vi "GEA2 Read and Update ERD.vi"(2 "Read Timeout (ms)":u32=500, 3 "Retry Count":i32=5, 5 "GEA Inputs":T2 {"Destination" format="%.0x"; "Source" format="%.0x"}, 7 "ERD Number":u16 format="%.0x", 9 "Update Information":string, 11 "Error In":errorcluster, 13 "Verify ERD Response?":bool=TRUE) -> (6 "Updated Raw Data Out":string, 8 "Updated ERD Data Out":T1 {"ERD Number" format="%.0x"}, 15 "Error Out":errorcluster)   [LabVIEW 2016, in "GEA2_Toolkit.lvlib"]
doc: "This VI reads and updates a single ERD based on the information provided in the Update information input. This VI only supports ERDs that support read and write capability. The update information should contain all of the bits that you wish to be updated in the ERD. Just specify the bits you want to update (ex. 0=1) and put whether or not you want them to be True (1) or False (0). You can specify a range of bits by using the - command in between two numbers (ex. 0-7=1 would change bits 0, 1, 2, 3, 4, 5, 6, 7 to true). The update information is converted to an array of strings by a comma delimiter. So, seperate your update information pieces by commas (Ex. if you wanted to make bits 0 and 10 false you could use the message: 0=0,10=0). Make sure you don't set the same bit twice or only the 2nd setting will ocurr (ex. 0=1,0=0 will only set bit 0 to false). If you were to write the following ERD data (00 01 02), byte 00 would be the byte 0 and contain bits 0-7, byte 01 would be byte 1 and contain bits 8-15, and byte 02 would be byte 2 and contain bits 16-23. For all bytes, the right-most bit is the first bit and the left-most bit is the last (Ex. For byte 00 being the hex value 0x01, bit 0 would be equal to 1 and would be the right-most bit (00000001)."
uses:
  library/GEA2_Toolkit.lvlib
  type defs/Source_Destination.ctl
  type defs/ERD Read Data Out.ctl
  C:/Technology Lab/NI-2010/Trunk/Utility/LabVIEW GEA2 Toolkit v1.0.0.0/Appliance.NET/GeaCommunication.dll
  Appliance.NET/GeaCommunication.dll
  type defs/ERD Read Data In.ctl
  type defs/Data Type.ctl
  type defs/ERD Write Data In.ctl
panel:
  out "GEA2 Reference Out":refnum<k24>
  in  "GEA2 Reference In":refnum<k24>
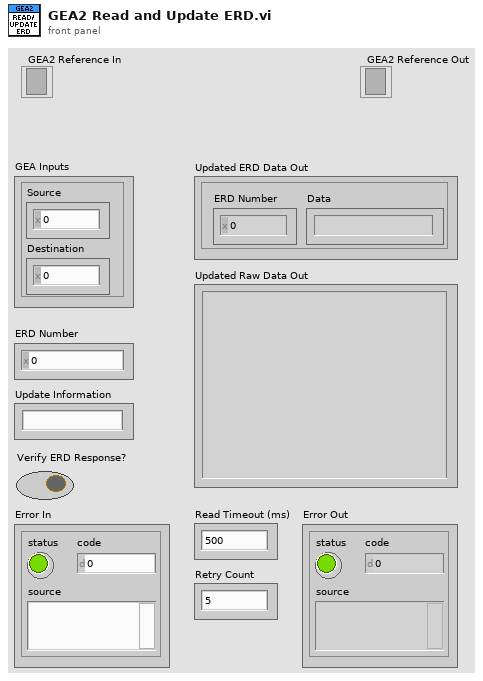
[diagram p1: front panel]
types:
  T1 = typedef "GEA2_Toolkit.lvlib/ERD Read Data Out.ctl" = cluster{"ERD Number":u16, "Data":string}
  T2 = typedef "GEA2_Toolkit.lvlib/Source_Destination.ctl" = cluster{"Source":u8, "Destination":u8}
  T3 = typedef "GEA2_Toolkit.lvlib/ERD Write Data In.ctl" = cluster{"ERD Number":u16, "Data Type":T4, "Data":string}
  T4 = typedef "GEA2_Toolkit.lvlib/Data Type.ctl" = enum16{"string", "boolean", "uint8_t", "uint16_t", "uint32_t", "uint64_t"}
  T5 = typedef "GEA2_Toolkit.lvlib/ERD Read Data In.ctl" = cluster{"ERD Number":u16, "Data Type":T4}
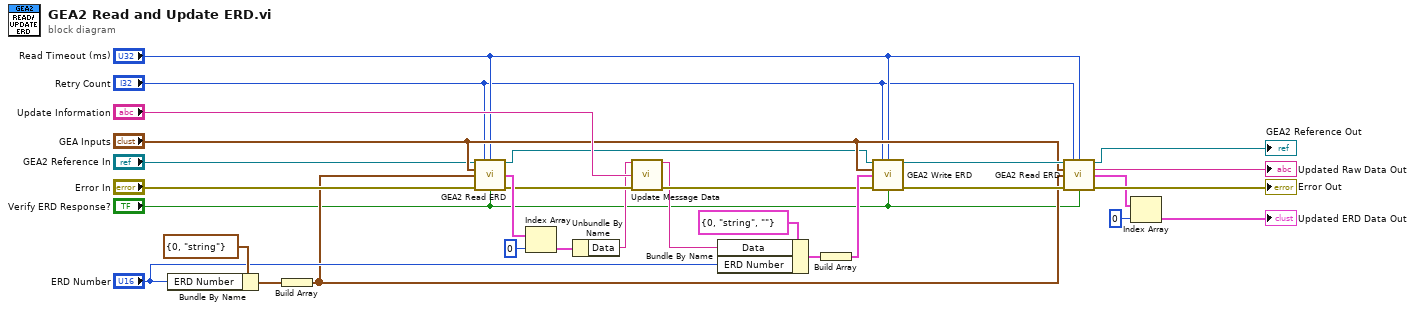
[diagram p0: block diagram]
diagram:
  n1 = Bundle By Name(cluster=T5 {"ERD Number"=0, "Data Type"=enum."string"} ("ERD Read Data In"), "ERD Number"="ERD Number") -> (w29:T5)
  n2 = Build Array(w29) -> (w12:T5[])
  n3 = call "GEA2 Read ERD.vi"("GEA2 Reference In"="GEA2 Reference In", "Retry Count"="Retry Count", "Read Timeout (ms)"="Read Timeout (ms)", "GEA Inputs"="GEA Inputs", "Read ERD List"=w12, "Error In"="Error In", "Verify ERD Response?"="Verify ERD Response?") -> ("GEA2 Reference Out"=w9:refnum<k24>, "ERD Data Out"=w27:T1[], "Error Out"=w17:errorcluster)  [unwired: 4 in, 2 out]
  n4 = Index Array(array=w27, index=0) -> (element=w25:T1)
  n5 = Unbundle By Name(w25) -> ("Data"=w14:string)
  n6 = call "Update Message Data.vi"("Data In"=w14, "Update Information"="Update Information", "Error In"=w17) -> ("Data Out"=w13:string, "Error Out"=w16:errorcluster)  [unwired: 11 in]
  n7 = Bundle By Name(cluster=T3 {"ERD Number"=0, "Data Type"=enum."string", "Data"=""} ("ERD Read Data In"), "Data"=w13, "ERD Number"="ERD Number") -> (w22:T3)
  n8 = Build Array(w22) -> (w21:T3[])
  n9 = call "GEA2 Write ERD.vi"("GEA2 Reference In"=w9, "Retry Count"="Retry Count", "Read Timeout (ms)"="Read Timeout (ms)", "GEA Inputs"="GEA Inputs", "Write ERD List"=w21, "Error In"=w16, "Verify ERD Response?"="Verify ERD Response?") -> ("GEA2 Reference Out"=w19:refnum<k24>, "Error Out"=w20:errorcluster)  [unwired: 6 in, 1 out]
  n10 = call "GEA2 Read ERD.vi"("GEA2 Reference In"=w19, "Retry Count"="Retry Count", "Read Timeout (ms)"="Read Timeout (ms)", "GEA Inputs"="GEA Inputs", "Read ERD List"=w12, "Error In"=w20, "Verify ERD Response?"="Verify ERD Response?") -> ("GEA2 Reference Out"=→"GEA2 Reference Out":refnum<k24>, "Raw Data Out"=→"Updated Raw Data Out":string, "ERD Data Out"=w6:T1[], "Error Out"=→"Error Out":errorcluster)  [unwired: 4 in, 1 out]
  n11 = Index Array(array=w6, index=0) -> (element=→"Updated ERD Data Out":T1)
